vi "Cell V Set.vi"(7 "Box ID":u8, 8 "error in (no error)":errorcluster, 9 "Voltage":dbl, 10 "Channel":u16, 11 "ENET in":refnum<class "ENET_BS120x.lvclass">) -> (0 "error out":errorcluster, 3 "ENET out":refnum<class "ENET_BS120x.lvclass">)   [LabVIEW 2021, in "BS120x Driver.lvlib" / "ENET_BS120x.lvclass"]
uses:
  ENET_BS120x.lvclass
  BS120x.lvclass
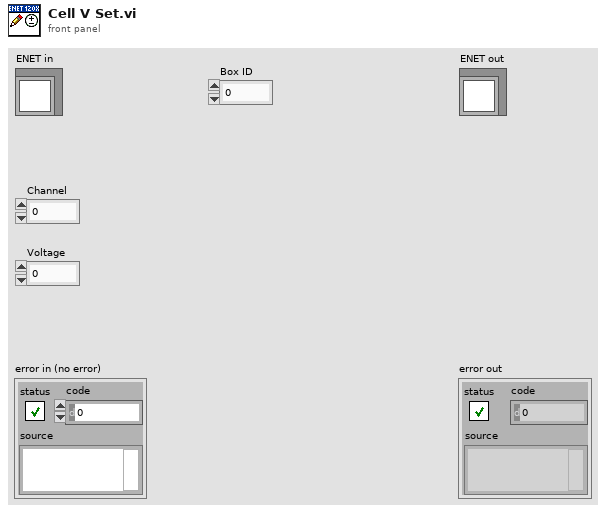
[diagram p1: front panel]
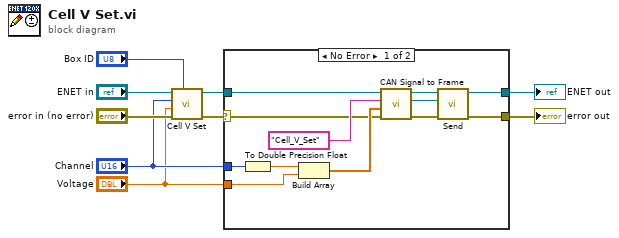
[diagram p0: block diagram]
diagram:
  n1 = call-parent "Cell V Set.vi"("Box ID"="Box ID", "error in (no error)"="error in (no error)", "Voltage"="Voltage", "Channel"="Channel", "BS120x in"="ENET in") -> ("error out"=w3:errorcluster, "BS120x out"=w6:refnum<class "ENET_BS120x.lvclass">)  [unwired: 5 in]
  n2 = case shown="No Error" w3 {
    selector: w3 -> [w11 w22]
    tunnel: [w17 w22] -> w9
    tunnel: "Voltage" -> [w10 _]
    tunnel: [w14 w23] -> w7
    tunnel: w6 -> [w13 w23]
    tunnel: "Channel" -> [w12 _]
    frame No Error {
      n3 = To Double Precision Float(number=w12) -> (double precision float=w16:dbl)
      n4 = Build Array(w16, w10) -> (w15:dbl[])
      n5 = call "CAN Signal to Frame.vi"("error in (no error)"=w11, "Data Array"=w15, "Frame"="Cell_V_Set", "ENET in"=w13) -> ("error out"=w18:errorcluster, "Data"=w19:refnum<class "Data.lvclass">, "ENET out"=w20:refnum<class "ENET_BS120x.lvclass">)  [unwired: 5 in]
      n6 = call "Send.vi"("error in (no error)"=w18, "Data"=w19, "ENET in"=w20) -> ("error out"=w17:errorcluster, "ENET out"=w14:refnum<class "ENET_BS120x.lvclass">)  [unwired: 7 in]
    }
    frame Error {
    }
  }
  "error out" <- w9
  "ENET out" <- w7
